vi "3.11--Genereate Function.vi"(1 "Left Data":T1, 2 "Right Data":T1) -> (0 "Function":dbl[](array[numeric]))   [LabVIEW 2011]
uses:
  4-High Neurons/4.1.2-Act Neuron TD.ctl
  3.0-Global.vi
panel:
  out "size(s)":i32
  out "XY Graph":cluster{dbl[], dbl[]}(graph)
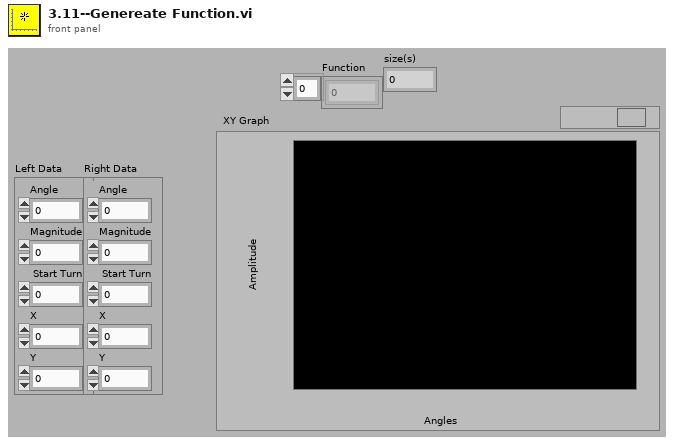
[diagram p1: front panel]
types:
  T1 = cluster{"Angle":dbl, "Magnitude":dbl, " Start Turn":dbl, "X":dbl, "Y":dbl}
  T2 = enum16{"Set Joystick", "Read Joystick", "Set Forebrain", "Read Forebrain", "Set Limbic", "Read Limbic", "Set Cerebellum", "Read Cerebellum", "Set Arbitrated", "Read Arbitrated", "Set LIDAR", "Read LIDAR", "Read Shallow Map", "Set Shallow Map"}
  T3 = typedef "4.1.2-Act Neuron TD.ctl" = cluster{"Speed By Path":sgl[]}
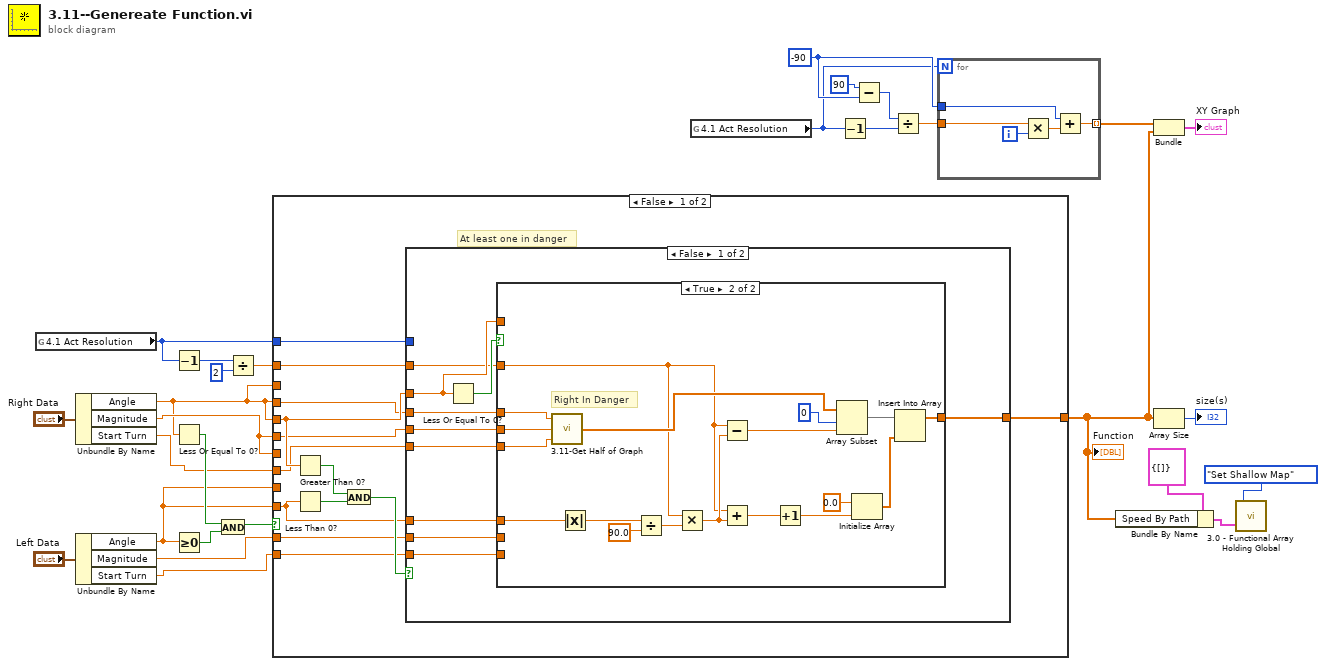
[diagram p0: block diagram]
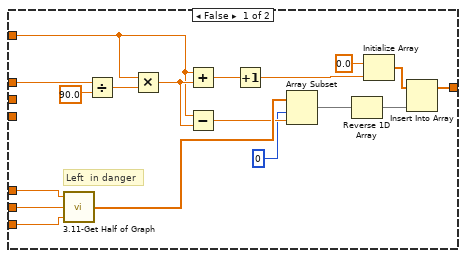
[diagram p2: hidden frame]
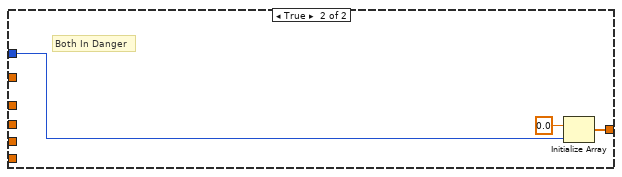
[diagram p3: hidden frame]
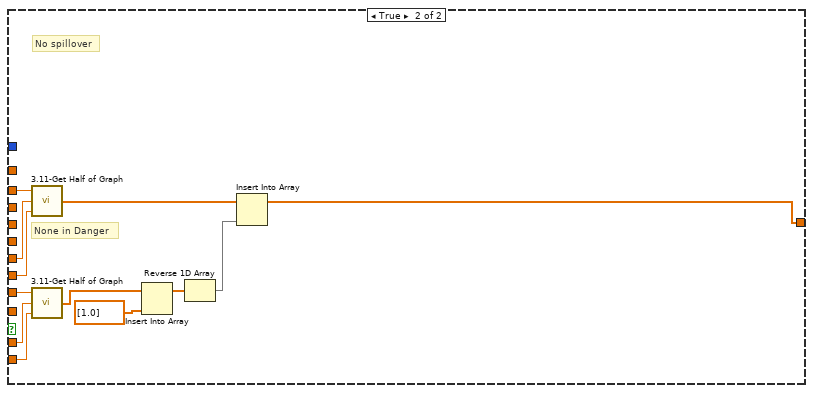
[diagram p4: hidden frame]
diagram:
  w24 = -90
  n1 = global read "3.0-Global.vi" "4.1 Act Resolution"() -> (w9:u32)
  n2 = Unbundle By Name("Right Data") -> ("Angle"=w7:dbl, "Magnitude"=w17:dbl, "Start Turn"=w8:dbl)
  n3 = Unbundle By Name("Left Data") -> ("Angle"=w6:dbl, "Magnitude"=w28:dbl, "Start Turn"=w5:dbl)
  n4 = Decrement(x=w9) -> (x-1=w10:u32)
  n5 = Less Or Equal To 0?(x=w7) -> (x <= 0?=w20:bool)
  n6 = Greater Or Equal To 0?(x=w6) -> (x >= 0?=w19:bool)
  n7 = And(x=w20, y=w19) -> (x .and. y?=w18:bool)
  n8 = Divide(x=w10, y=u32 2) -> (x/y=w11:dbl)
  n9 = case shown="False" w18 {
    tunnel: w28 -> [w32 w102]
    tunnel: [w38 w101] -> w3
    tunnel: w6 -> [_ w100]
    tunnel: w5 -> [w34 w99]
    tunnel: w7 -> [_ w98]
    tunnel: w17 -> [_ w97]
    tunnel: w8 -> [w31 w96]
    tunnel: w6 -> [w36 _]
    tunnel: w7 -> [w37 _]
    tunnel: w7 -> [w35 _]
    tunnel: w17 -> [w33 _]
    tunnel: w11 -> [w30 _]
    tunnel: w9 -> [w29 _]
    frame False {
      # "At least one in danger"
      n10 = Greater Than 0?(x=w37) -> (x > 0?=w40:bool)
      n11 = Less Than 0?(x=w36) -> (x < 0?=w41:bool)
      n12 = And(x=w40, y=w41) -> (x .and. y?=w39:bool)
      n13 = case shown="False" w39 {
        tunnel: [w43 w89] -> w38
        tunnel: w37 -> [w50 _]
        tunnel: w36 -> [w47 _]
        tunnel: w35 -> [w49 _]
        tunnel: w34 -> [w48 _]
        tunnel: w33 -> [w46 _]
        tunnel: w32 -> [w45 _]
        tunnel: w31 -> [w44 _]
        tunnel: w30 -> [w42 _]
        tunnel: w29 -> [_ w88]
        frame False {
          n14 = Less Or Equal To 0?(x=w50) -> (x <= 0?=w51:bool)
          n15 = case shown="True" w51 {
            tunnel: w50 -> [_ _]
            tunnel: w49 -> [w69 w80]
            tunnel: w48 -> [w62 _]
            tunnel: w47 -> [w64 w81]
            tunnel: w46 -> [_ w79]
            tunnel: w45 -> [w63 _]
            tunnel: w44 -> [_ w78]
            tunnel: [w58 w75] -> w43
            tunnel: w42 -> [w52 w70]
            frame False {
              # "Left  in danger"
              n16 = call "3.11-Get Half of Graph.vi"("Start Turn"=w62, "Magnitude"=w63, "Angle"=w64) -> ("Array"=w60:dbl[])
              n17 = Divide(x=w69, y=90.0) -> (x/y=w67:dbl)
              n18 = Multiply(x=w52, y=w67) -> (x*y=w57:dbl)
              n19 = Add(x=w52, y=w57) -> (x+y=w59:dbl)
              n20 = Subtract(x=w52, y=w57) -> (x-y=w55:dbl)
              n21 = Increment(x=w59) -> (x+1=w65:dbl)
              n22 = Array Subset(array=w60, index=0, length=w55) -> (w56:dbl[])
              n23 = Reverse 1D Array(array=w56) -> (reversed array=w53:dbl[])
              n24 = Initialize Array(0.0 ("element"), w65) -> (w61:dbl[])
              n25 = Insert Into Array(array=w61, new element=w53) -> (w58:dbl[])  [unwired: 1 in]
            }
            frame True {
              # "Right In Danger"
              n26 = call "3.11-Get Half of Graph.vi"("Start Turn"=w78, "Magnitude"=w79, "Angle"=w80) -> ("Array"=w83:dbl[])
              n27 = Absolute Value(x=w81) -> (abs(x)=w74:dbl)
              n28 = Divide(x=w74, y=90.0) -> (x/y=w86:dbl)
              n29 = Multiply(x=w70, y=w86) -> (x*y=w71:dbl)
              n30 = Subtract(x=w70, y=w71) -> (x-y=w72:dbl)
              n31 = Add(x=w70, y=w71) -> (x+y=w82:dbl)
              n32 = Increment(x=w82) -> (x+1=w84:dbl)
              n33 = Array Subset(array=w83, index=0, length=w72) -> (w77:dbl[])
              n34 = Initialize Array(0.0 ("element"), w84) -> (w76:dbl[])
              n35 = Insert Into Array(array=w77, new element=w76) -> (w75:dbl[])  [unwired: 1 in]
            }
          }
        }
        frame True {
          # "Both In Danger"
          n36 = Initialize Array(0.0 ("element"), w88) -> (w89:dbl[])
        }
      }
    }
    frame True {
      # "None in Danger"
      # "No spillover"
      n37 = call "3.11-Get Half of Graph.vi"("Start Turn"=w96, "Magnitude"=w97, "Angle"=w98) -> ("Array"=w91:dbl[])
      n38 = call "3.11-Get Half of Graph.vi"("Start Turn"=w99, "Magnitude"=w102, "Angle"=w100) -> ("Array"=w95:dbl[])
      n39 = Insert Into Array(array=w95, new element=dbl[] [1.0] ("array")) -> (w93:dbl[])  [unwired: 1 in]
      n40 = Reverse 1D Array(array=w93) -> (reversed array=w92:dbl[])
      n41 = Insert Into Array(array=w91, new element=w92) -> (w101:dbl[])  [unwired: 1 in]
    }
  }
  "Function" <- w3
  n42 = global read "3.0-Global.vi" "4.1 Act Resolution"() -> (w13:u32)
  n43 = Decrement(x=w13) -> (x-1=w23:u32)
  n44 = Subtract(x=90, y=w24) -> (x-y=w27:i32)
  n45 = Divide(x=w27, y=w23) -> (x/y=w26:dbl)
  n46 = for {
    N: w13 -> [_]
    tunnel: w26 -> [w106]
    tunnel: w24 -> [w104]
    tunnel: [w103] -> w22 mode=indexing
    i -> [w107]
    n47 = Multiply(x=w106, y=w107) -> (x*y=w105:dbl)
    n48 = Add(x=w104, y=w105) -> (x+y=w103:dbl)
  }
  n49 = Bundle By Name(cluster=T3 {"Speed By Path"=[]} ("Input Act Neurons"), "Speed By Path"=w3) -> (w2:T3)
  n50 = Bundle(w22, "Array"=w3) -> (→"XY Graph":cluster{dbl[], "Array":dbl[]})  [unwired: 1 in]
  n51 = Array Size(array=w3) -> (size(s)=→"size(s)":i32)
  n52 = call "3.0 - Functional Array Holding Global.vi"("Input Act Neurons"=w2, "Mode"=T2."Set Shallow Map") -> ()  [unwired: 1 out]
